vi "Set Bandwidth.vi"(9 "Bandwidth":u16(ring)=10 items=["1 kHz"=1, "5 kHz"=5, "10 kHz"=10, "25 kHz"=25, "50 kHz"=50, "100 kHz"=100], 11 "RS232":refnum<visa-resource-name>="ASRL27::INSTR") -> (0 "Success?":bool, 3 "RS232 out":refnum<visa-resource-name>="ASRL27::INSTR")   [LabVIEW 2022 SP3]
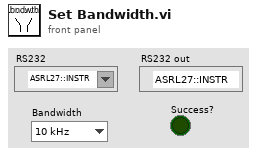
[diagram p1: front panel]
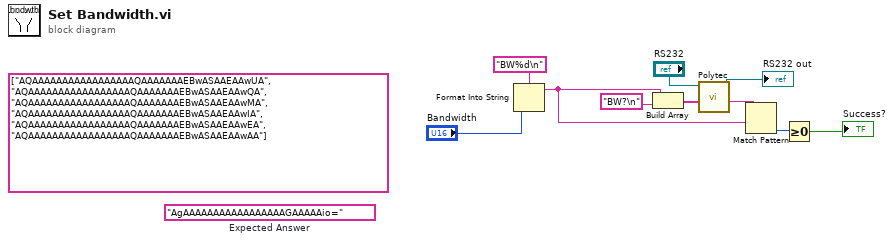
[diagram p0: block diagram]
diagram:
  (unwired) string[] ["AQAAAAAAAAAAAAAAAAAQAAAAAAAEBwASAAEAAwUA", "AQAAAAAAAAAAAAAAAAAQAAAAAAAEBwASAAEAAwQA", "AQAAAAAAAAAAAAAAAAAQAAAAAAAEBwASAAEAAwMA", "AQAAAAAAAAAAAAAAAAAQAAAAAAAEBwASAAEAAwIA", "AQAAAAAAAAAAAAAAAAAQAAAAAAAEBwASAAEAAwEA", "AQAAAAAAAAAAAAAAAAAQAAAAAAAEBwASAAEAAwAA"]
  (unwired) "AgAAAAAAAAAAAAAAAAAGAAAAAio="  # Expected Answer
  n1 = Format Into String(format string="BW%d\n", "Bandwidth") -> (resulting string=w1:string)  [unwired: 2 in, 1 out]
  n2 = Build Array(w1, "BW?\n" ("format string")) -> (w2:string[])
  n3 = call "Polytec.vi"("RS232"="RS232", "Strings"=w2) -> ("RS232 out"=→"RS232 out":refnum<visa-resource-name>, "String Read"=w8:string)  [unwired: 7 in]
  n4 = Match Pattern(string=w8, regular expression=w1) -> (offset past match=w9:i32)  [unwired: 1 in, 3 out]
  n5 = Greater Or Equal To 0?(x=w9) -> (x >= 0?=→"Success?":bool)
